vi "ini.vi"(8 "error in (no error)":errorcluster, 11 "LNAX301 in":refnum<class "LNAX301.lvclass">) -> (0 "error out":errorcluster, 3 "LNAX301 out":refnum<class "LNAX301.lvclass">)   [LabVIEW 2017, in "LNAX301.lvclass"]
uses:
  LNAX301.lvclass
  LNAX301.lvclass/LNAX301.ctl
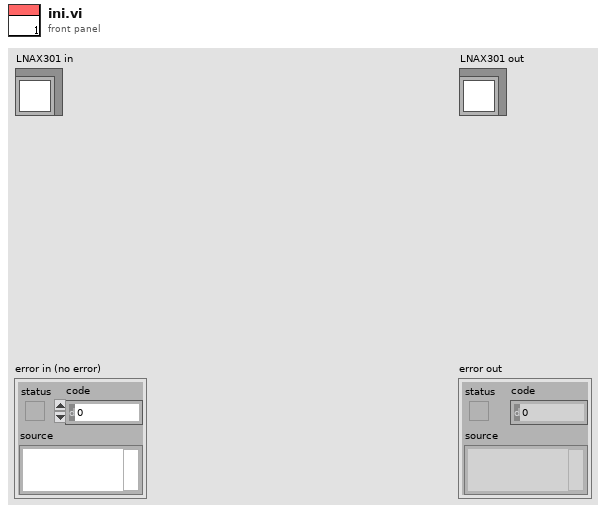
[diagram p1: front panel]
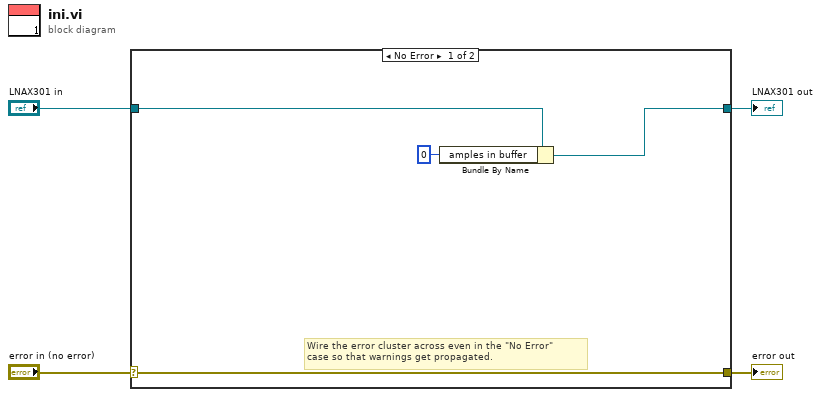
[diagram p0: block diagram]
diagram:
  n1 = case shown="No Error" "error in (no error)" {
    selector: "error in (no error)" -> [w8 w10]
    tunnel: [w8 w10] -> w3
    tunnel: [w6 w9] -> w1
    tunnel: "LNAX301 in" -> [w7 w9]
    frame No Error {
      # "Wire the error cluster across even in the \"No Error\"\ncase so that warnings get propagated."
      n2 = Bundle By Name(cluster=w7, "amples in buffer"=u16 0) -> (w6:refnum<class "LNAX301.lvclass">)
    }
    frame Error {
    }
  }
  "error out" <- w3
  "LNAX301 out" <- w1
